vi "constructor.vi"(0 "Line in":refnum<class "Line.lvclass">, 1 "Color Vector":sgl[](array[numeric]), 5 "X Vector":sgl[](array[numeric]), 7 "Y Vector":sgl[](array[numeric]), 9 "Z Vector":sgl[](array[numeric]), 11 "error in (no error)":errorcluster, 12 "Plot ID":i32) -> (4 "Line out":refnum<class "Line.lvclass">, 15 "error out":errorcluster)   [LabVIEW 2020, in "Line.lvclass"]
uses:
  <vilib>/Native 3D Graph/classes/Line/Line.lvclass
  <vilib>/Native 3D Graph/classes/Line/Line.lvclass/Line.ctl
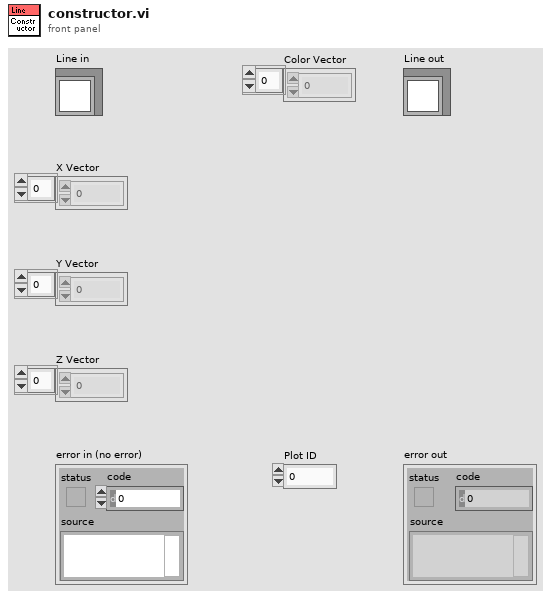
[diagram p1: front panel]
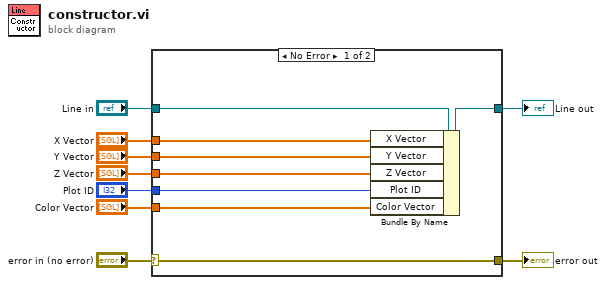
[diagram p0: block diagram]
diagram:
  n1 = case shown="No Error" "error in (no error)" {
    selector: "error in (no error)" -> [w17 w19]
    tunnel: [w17 w19] -> w8
    tunnel: [w15 w18] -> w6
    tunnel: "Line in" -> [w16 w18]
    tunnel: "Color Vector" -> [w14 _]
    tunnel: "Z Vector" -> [w13 _]
    tunnel: "Y Vector" -> [w12 _]
    tunnel: "X Vector" -> [w11 _]
    tunnel: "Plot ID" -> [w10 _]
    frame No Error {
      n2 = Bundle By Name(cluster=w16, "X Vector"=w11, "Y Vector"=w12, "Z Vector"=w13, "Plot ID"=w10, "Color Vector"=w14) -> (w15:refnum<class "Line.lvclass">)
    }
    frame Error {
    }
  }
  "error out" <- w8
  "Line out" <- w6
